vi "H5Lget_val_by_idx (Basic).vi"(5 "Order":T1 items=["H5_ITER_UNKNOWN"=-1, "H5_ITER_INC"=0, "H5_ITER_DEC"=1], 6 "lapl_id":T4, 7 "Index Field":T2 items=["H5_INDEX_UNKNOWN"=-1, "H5_INDEX_NAME"=0, "H5_INDEX_CRT_ORDER"=1], 8 "error in (no error)":errorcluster, 9 "Index":u64, 10 "Name":string=".", 11 "Location Ref":T4) -> (0 "error out":errorcluster, 1 "buffer":u8[](array[numeric]), 3 "Location Ref out":T4, 4 "type":T3 items=["H5L_TYPE_ERROR"=-1, "H5L_TYPE_HARD"=0, "H5L_TYPE_SOFT"=1, "H5L_TYPE_EXTERNAL"=64, "H5L_TYPE_MAX"=255])   [LabVIEW 2017]
doc: "Retrieves value of the nth link in a group, according to the order within an index."
uses:
  <vilib>/UPVI/lvhdf5/library.llb/HDF5 Ref.ctl
  <vilib>/UPVI/lvhdf5/link.llb/H5L_type_t.ctl
  <vilib>/UPVI/lvhdf5/library.llb/H5_index_t.ctl
  <vilib>/UPVI/lvhdf5/library.llb/H5_iter_order_t.ctl
  <vilib>/UPVI/lvhdf5/error.llb/LVH5EMajorID.ctl
  <vilib>/UPVI/lvhdf5/error.llb/LVH5EMinorID.ctl
  <vilib>/UPVI/lvhdf5/error.llb/H5Epush_enum_enum.vi
  <vilib>/UPVI/lvhdf5/hdf5.dll
panel:
  # "LVHDF5 Toolkit\nCopyright (c) 2005-2013 by Jason D. Sommerville\nCopyright (c) 2014-2015 by UPVI, LLC.\n\nThis use and distribution of this file is governed by the terms found in \nLICENSE.txt distributed with this toolkit and installed at\n <user.lib>\\_lvhdf5\\LICENSE.txt"
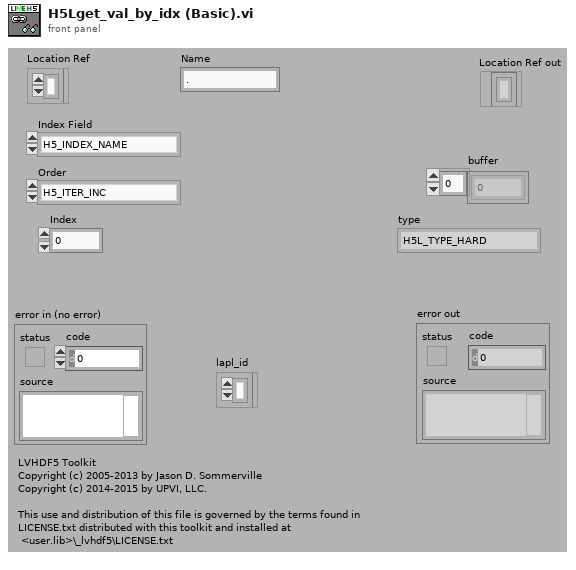
[diagram p1: front panel]
types:
  T1 = typedef "H5_iter_order_t.ctl" = i32
  T2 = typedef "H5_index_t.ctl" = i32
  T3 = typedef "H5L_type_t.ctl" = i32
  T4 = typedef "HDF5 Ref.ctl" = refnum<k1>
  T5 = typedef "LVH5EMinorID.ctl" = string
  T6 = typedef "LVH5EMajorID.ctl" = string
  T7 = typedef "H5L_info_t.ctl" = cluster{"type":T3, "corder_valid":bool, "corder":i64, "cset":T8, "address/val_size":u64}
  T8 = typedef "H5T_cset_t.ctl" = i32
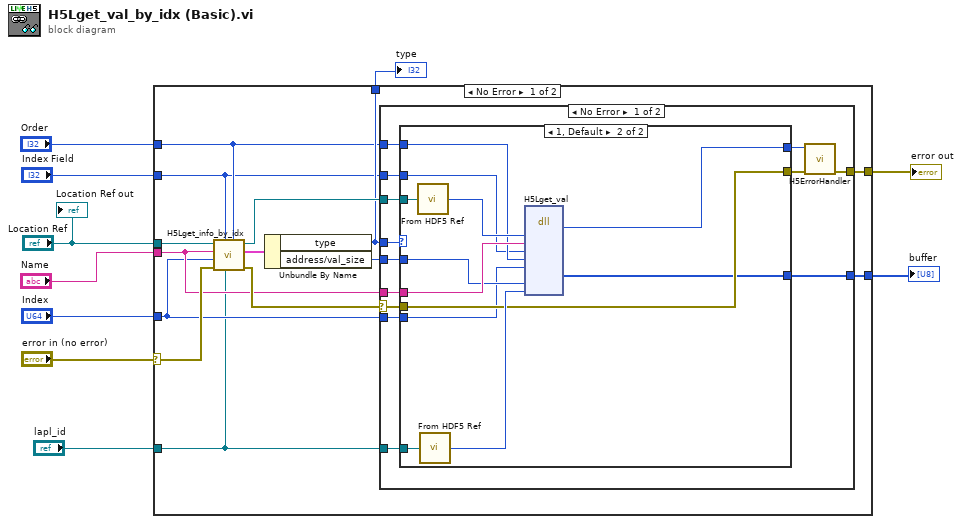
[diagram p0: block diagram]
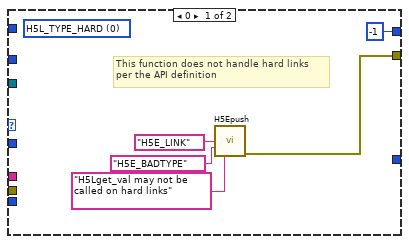
[diagram p2: hidden frame]
diagram:
  n1 = case shown="No Error" "error in (no error)" {
    selector: "error in (no error)" -> [w22 w55]
    tunnel: [w24 w55] -> w9
    tunnel: "lapl_id" -> [w11 _]
    tunnel: "Location Ref" -> [w23 _]
    tunnel: "Name" -> [w17 _]
    tunnel: [w16 _] -> w5
    tunnel: [w15 _] -> w4
    tunnel: "Index Field" -> [w13 _]
    tunnel: "Order" -> [w14 _]
    tunnel: "Index" -> [w12 _]
    frame No Error {
      n2 = call <vilib>:"H5Lget_info_by_idx.vi"("Order"=w14, "lapl_id"=w11, "Index Field"=w13, "error in (no error)"=w22, "Index"=w12, "Group Name"=w17, "Location Ref"=w23) -> ("error out"=w20:errorcluster, "H5L_info_t"=w21:T7, "Location Ref out"=w19:T4)  [unwired: 2 in]
      n3 = Unbundle By Name(w21) -> ("type"=w15:T3, "address/val_size"=w18:u64)
      n4 = case shown="No Error" w20 {
        selector: w20 -> [w32 w54]
        tunnel: [w36 w54] -> w24
        tunnel: w15 -> [w35 _]
        tunnel: w19 -> [w34 _]
        tunnel: w18 -> [w33 _]
        tunnel: w17 -> [w31 _]
        tunnel: w11 -> [w30 _]
        tunnel: [w28 _] -> w16
        tunnel: w14 -> [w27 _]
        tunnel: w13 -> [w26 _]
        tunnel: w12 -> [w25 _]
        frame No Error {
          n5 = case shown="1, Default" w35 {
            tunnel: [w38 w46] -> w36
            tunnel: w34 -> [_ w53]
            tunnel: w33 -> [_ w50]
            tunnel: w32 -> [_ w46]
            tunnel: w31 -> [_ w51]
            tunnel: w30 -> [_ w49]
            tunnel: [-1 ("return type") w47] -> w29
            tunnel: [_ w45] -> w28
            tunnel: w27 -> [_ w44]
            tunnel: w26 -> [_ w43]
            tunnel: w25 -> [_ w42]
            frame 0 {
              (unwired) T3 0 items=["H5L_TYPE_ERROR"=-1, "H5L_TYPE_HARD"=0, "H5L_TYPE_SOFT"=1, "H5L_TYPE_EXTERNAL"=64, "H5L_TYPE_MAX"=255] ("type")
              # "This function does not handle hard links\nper the API definition"
              n6 = call-poly <vilib>:"H5Epush.vi"("major_id"=T6 "H5E_LINK", "minor_id"=T5 "H5E_BADTYPE", "msg"="H5Lget_val may not be called on hard links") -> ("error out"=w38:errorcluster)  [unwired: 11 in, 1 out]
            }
            frame 1, Default {
              n7 = call <vilib>:"From HDF5 Ref.vi"("HDF5 Ref"=w53) -> ("I32"=w52:i32)
              n8 = call <vilib>:"From HDF5 Ref.vi"("HDF5 Ref"=w49) -> ("I32"=w48:i32)
              n9 = dll-call lib="C:/Program Files/National Instruments/LabVIEW 2017/vi.lib/UPVI/lvhdf5/hdf5.dll" fn="H5Lget_val" label="H5Lget_val_by_idx"("loc_id"=w52, "name"=w51, "index_type"=w43, "order"=w44, "n"=w42, "size"=w50, "lapl_id"=w48) -> ("return type"=w47:i32, "buff"=w45:u8[])  [unwired: 11 in, 2 out]
            }
          }
          n10 = call <vilib>:"H5ErrorHandler.vi"("herr_t"=w29) -> ()  [unwired: 4 in, 5 out]
        }
        frame Error {
        }
      }
    }
    frame Error {
    }
  }
  "error out" <- w9
  "buffer" <- w5
  "type" <- w4
  "Location Ref out" <- "Location Ref"
